vi "Update.vi"(4 "Value2":dbl, 6 "Value1":dbl, 8 "error in (no error)":errorcluster, 9 "Audio History Buffer In":dbl[][](array[numeric]), 10 "Audio Data In":dbl[][](array[numeric]), 11 "Flanger in":refnum<class "Flanger.lvclass">) -> (0 "error out":errorcluster, 1 "Audio History Buffer Out":dbl[][](array[numeric]), 2 "Audio Data Out":dbl[][](array[numeric]), 3 "Flanger out":refnum<class "Flanger.lvclass">)   [LabVIEW 2019, in "Flanger.lvlib" / "Flanger.lvclass"]
doc: "Applies the flanger effect. The effect is produced by adding a duplicate audio signal to the original, with a slowly shifting phase.\n\n<b>Value1:</b> Dry/wet amount\n<b>Value2:</b> Phase shift frequency"
uses:
  Flanger.lvclass
  Flanger.lvclass/Flanger.ctl
  <vilib>/ptbypt/NI_PtbyPt.lvlib
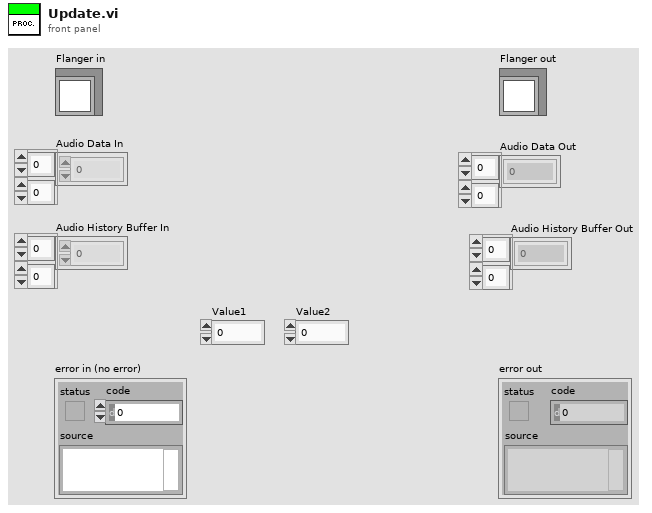
[diagram p1: front panel]
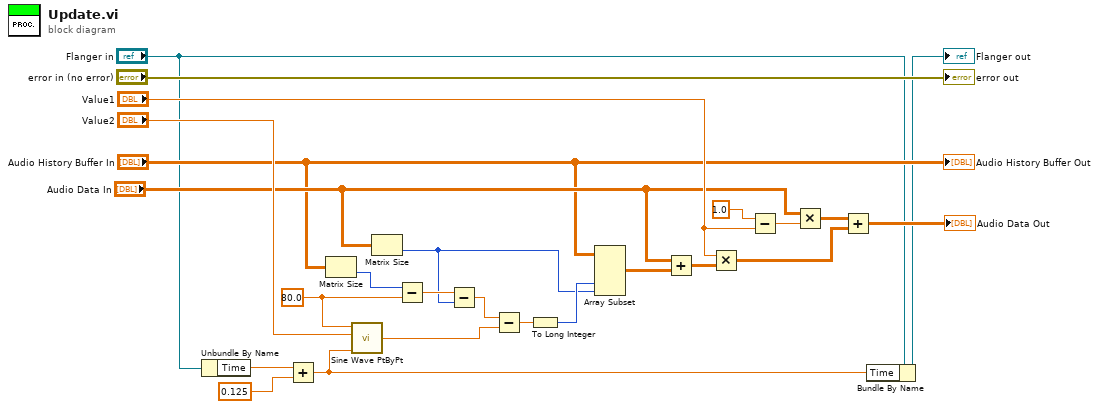
[diagram p0: block diagram]
diagram:
  w16 = 80.0 ("Delay")
  n1 = Unbundle By Name("Flanger in") -> ("Time"=w4:dbl)
  n2 = Add(x=w4, y=0.125) -> (x+y=w1:dbl)
  n3 = Matrix Size(0:"Audio History Buffer In") -> (2:w11:i32)  [unwired: 1 out]
  n4 = call <vilib>:"Sine Wave PtByPt.vi"("time"=w1, "frequency"="Value2", "amplitude"=w16) -> ("sine wave"=w13:dbl)  [unwired: 1 in]
  n5 = Matrix Size(0:"Audio Data In") -> (2:w12:i32)  [unwired: 1 out]
  n6 = Subtract(x=w11, y=w16) -> (x-y=w17:dbl)
  n7 = Subtract(x=w17, y=w12) -> (x-y=w18:dbl)
  n8 = Subtract(x=w18, y=w13) -> (x-y=w14:dbl)
  n9 = To Long Integer(number=w14) -> (32bit integer=w15:i32)
  n10 = Array Subset(array="Audio History Buffer In", index (col)=w15, length (col)=w12) -> (w25:dbl[][])  [unwired: 2 in]
  n11 = Add(x="Audio Data In", y=w25) -> (x+y=w20:dbl[][])
  n12 = Multiply(x="Value1", y=w20) -> (x*y=w24:dbl[][])
  n13 = Subtract(x=1.0, y="Value1") -> (x-y=w22:dbl)
  n14 = Multiply(x="Audio Data In", y=w22) -> (x*y=w23:dbl[][])
  n15 = Add(x=w23, y=w24) -> (x+y=→"Audio Data Out":dbl[][])
  n16 = Bundle By Name(cluster="Flanger in", "Time"=w1) -> (→"Flanger out":refnum<class "Flanger.lvclass">)
  "error out" <- "error in (no error)"
  "Audio History Buffer Out" <- "Audio History Buffer In"
